vi "Destroy.vi"(0 "reference in":refnum<class "J1939-22_Database.lvclass">, 5 "Error In":errorcluster) -> (14 "reference out":refnum<class "J1939-22_Database.lvclass">, 19 "Error Out":errorcluster)   [LabVIEW 2021, in "J1939-22_Database.lvclass"]
uses:
  J1939-22_Database.lvclass
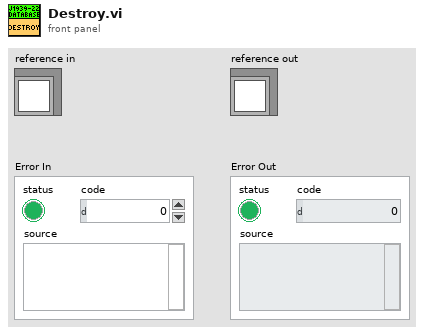
[diagram p1: front panel]
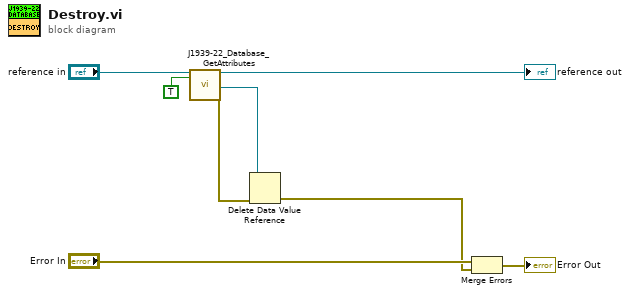
[diagram p0: block diagram]
diagram:
  n1 = call "J1939-22_Database_GetAttributes.vi"("reference in"="reference in", "OnlyGetDvrReference(False)"=TRUE) -> ("reference out"=→"reference out":refnum<class "J1939-22_Database.lvclass">, "DataRef"=w4:refnum<data-value>, "Error Out"=w5:errorcluster)  [unwired: 14 in, 1 out]
  n2 = Delete Data Value Reference(data value reference=w4, error in=w5) -> (error out=w2:errorcluster)  [unwired: 1 out]
  n3 = Merge Errors("Error In", w2) -> (→"Error Out":errorcluster)
